vi "recombine group data.vi"(8 "error in":errorcluster, 9 "specification":T1[](array[typedef]), 10 "group in":T3, 11 "data table in":T3) -> (0 "error out":errorcluster, 2 "group out":T3, 3 "data table out":T3)   [LabVIEW 2013, in "tag bus.lvlib" / "data table.lvlib"]
doc: "Accepts a primary data table and a subgroup data table, and copies data from the group into the main table."
uses:
  data table.lvlib
  data table.ctl
  group specification.ctl
  tag/Data Type.ctl
  data polymorphs/write many/write Doubles.vi
  data polymorphs/read all/read all Doubles.vi
  data polymorphs/write many/write Singles.vi
  data polymorphs/read all/read all Singles.vi
  data polymorphs/write many/write I64s.vi
  data polymorphs/read all/read all I64s.vi
  data polymorphs/write many/write I32s.vi
  data polymorphs/read all/read all I32s.vi
  data polymorphs/write many/write I16s.vi
  data polymorphs/read all/read all I16s.vi
  data polymorphs/write many/write I8s.vi
  data polymorphs/read all/read all I8s.vi
  data polymorphs/write many/write U64s.vi
  data polymorphs/read all/read all U64s.vi
  data polymorphs/write many/write U32s.vi
  data polymorphs/read all/read all U32s.vi
  data polymorphs/write many/write U16s.vi
  data polymorphs/read all/read all U16s.vi
  data polymorphs/write many/write U8s.vi
  data polymorphs/read all/read all U8s.vi
  data polymorphs/write many/write Strings.vi
  data polymorphs/read all/read all Strings.vi
  data polymorphs/write many/write Booleans.vi
  data polymorphs/read all/read all Booleans.vi
  data polymorphs/write many/write Array of U8s.vi
  data polymorphs/read all/read all Array of U8s.vi
  data polymorphs/write many/write Array of U16s.vi
  data polymorphs/read all/read all Array of U16s.vi
  data polymorphs/write many/write Array of U32s.vi
  data polymorphs/read all/read all Array of U32s.vi
  data polymorphs/write many/write Array of U64s.vi
  data polymorphs/read all/read all Array of U64s.vi
  data polymorphs/write many/write Array of I64s.vi
  data polymorphs/read all/read all Array of I64s.vi
  data polymorphs/write many/write Array of I32s.vi
  data polymorphs/read all/read all Array of I32s.vi
  data polymorphs/write many/write Array of I16s.vi
  data polymorphs/read all/read all Array of I16s.vi
  data polymorphs/write many/write Array of I8s.vi
  data polymorphs/read all/read all Array of I8s.vi
  data polymorphs/write many/write Array of Doubles.vi
  data polymorphs/read all/read all Array of Doubles.vi
  data polymorphs/write many/write Array of Singles.vi
  data polymorphs/read all/read all Array of Singles.vi
  data polymorphs/write many/write Array of Booleans.vi
  data polymorphs/read all/read all Array of Booleans.vi
  data polymorphs/write many/write Array of Strings.vi
  data polymorphs/read all/read all Array of Strings.vi
  tag/tag descriptor.lvclass
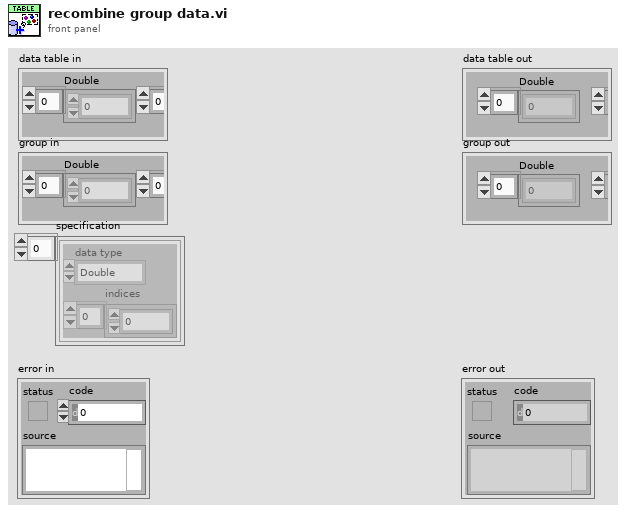
[diagram p1: front panel]
types:
  T1 = typedef "tag bus.lvlib/data table.lvlib/group specification.ctl" = cluster{"data type":T2, "indices":i32[]}
  T2 = typedef "tag bus.lvlib/tag descriptor.lvclass/Data Type.ctl" = enum16{"Double", "Single", "I64", "I32", "I16", "I8", "U64", "U32", "U16", "U8", "Boolean", "String", "Array of Double", "Array of Single", "Array of I64", "Array of I32", "Array of I16", "Array of I8", "Array of U64", "Array of U32", "Array of U16", "Array of U8", "Array of Boolean", "Array of String"}
  T3 = typedef "tag bus.lvlib/data table.lvlib/data table.ctl" = cluster{"Double":dbl[], "Single":sgl[], "I64":i64[], "I32":i32[], "I16":i16[], "I8":i8[], "U64":u64[], "U32":u32[], "U16":u16[], "U8":u8[], "Boolean":bool[], "String":string[], "Array of Double":cluster{"DBL Array":dbl[]}[], "Array of Single":cluster{"SGL Array":sgl[]}[], "Array of I64":cluster{"I64 Array":i64[]}[], "Array of I32":cluster{"I32 Array":i32[]}[], "Array of I16":cluster{"I16 Array":i16[]}[], "Array of I8":cluster{"I8 Array":i8[]}[], "Array of U64":cluster{"U64 Array":u64[]}[], "Array of U32":cluster{"U32 Array":u32[]}[], "Array of U16":cluster{"U16 Array":u16[]}[], "Array of U8":cluster{"U8 Array":u8[]}[], "Array of Boolean":cluster{"Boolean Array":bool[]}[], "Array of String":cluster{"String Array":string[]}[]}
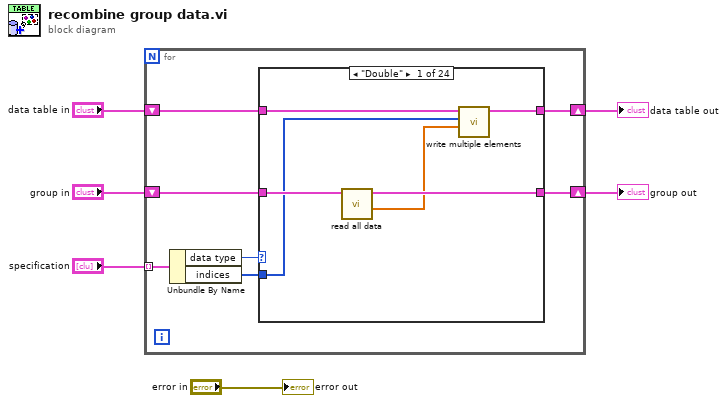
[diagram p0: block diagram]
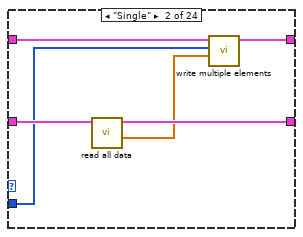
[diagram p2: hidden frame]
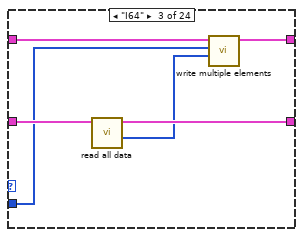
[diagram p3: hidden frame]
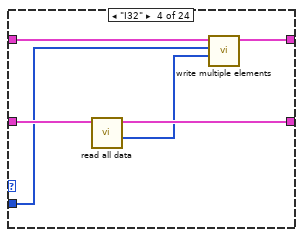
[diagram p4: hidden frame]
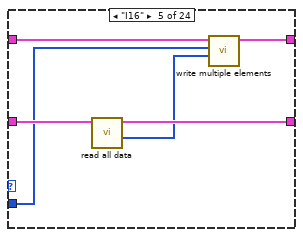
[diagram p5: hidden frame]
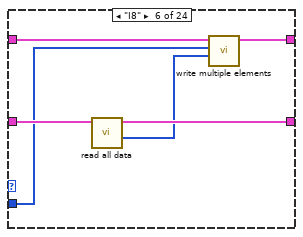
[diagram p6: hidden frame]
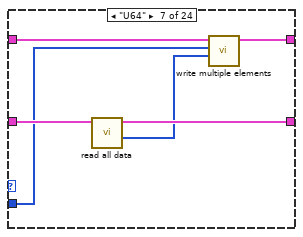
[diagram p7: hidden frame]
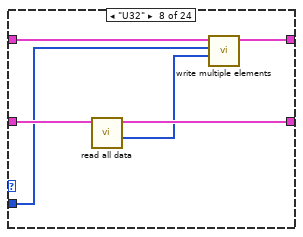
[diagram p8: hidden frame]
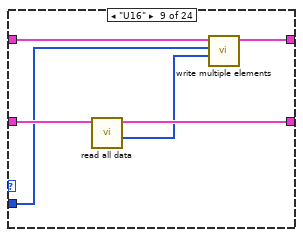
[diagram p9: hidden frame]
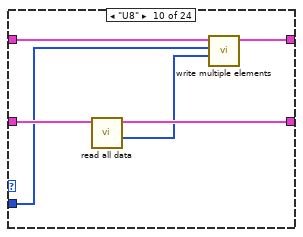
[diagram p10: hidden frame]
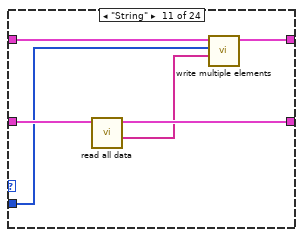
[diagram p11: hidden frame]
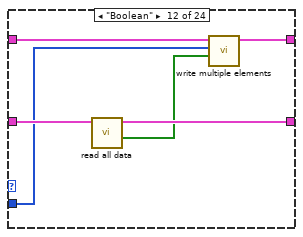
[diagram p12: hidden frame]
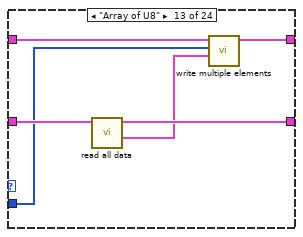
[diagram p13: hidden frame]
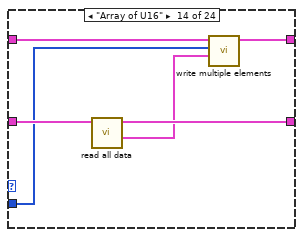
[diagram p14: hidden frame]
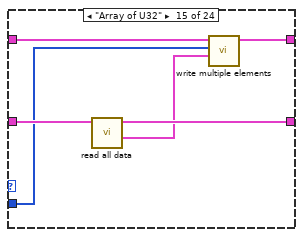
[diagram p15: hidden frame]
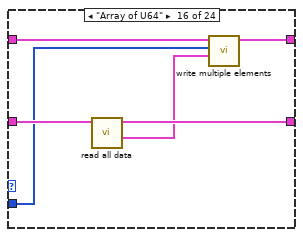
[diagram p16: hidden frame]
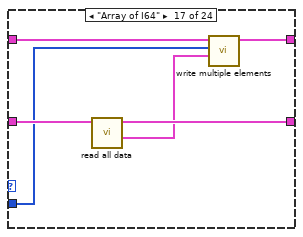
[diagram p17: hidden frame]
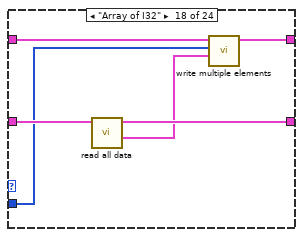
[diagram p18: hidden frame]
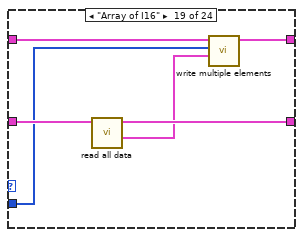
[diagram p19: hidden frame]
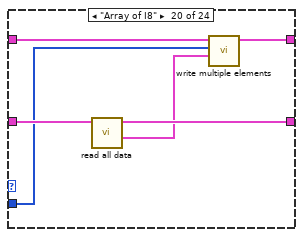
[diagram p20: hidden frame]
diagram:
  n1 = for {
    shift-right: [w9] -> w5
    shift-left: "data table in" -> [w10]
    shift-right: [w7] -> w3
    shift-left: "group in" -> [w8]
    tunnel: "specification" -> [w13] mode=indexing
    n2 = Unbundle By Name(w13) -> ("data type"=w12:T2, "indices"=w11:i32[])
    n3 = case shown="\"Double\"" w12 {
      tunnel: w11 -> [w14 w20 w26 w32 w38 w44 w50 w56 w62 w68 w74 w80 w86 w92 w98 w104 w110 w116 w122 w128 w134 w140 w146 w152]
      tunnel: w10 -> [w16 w22 w28 w34 w40 w46 w52 w58 w64 w70 w76 w82 w88 w94 w100 w106 w112 w118 w124 w130 w136 w142 w148 w154]
      tunnel: [w15 w21 w27 w33 w39 w45 w51 w57 w63 w69 w75 w81 w87 w93 w99 w105 w111 w117 w123 w129 w135 w141 w147 w153] -> w9
      tunnel: w8 -> [w19 w25 w31 w37 w43 w49 w55 w61 w67 w73 w79 w85 w91 w97 w103 w109 w115 w121 w127 w133 w139 w145 w151 w157]
      tunnel: [w18 w24 w30 w36 w42 w48 w54 w60 w66 w72 w78 w84 w90 w96 w102 w108 w114 w120 w126 w132 w138 w144 w150 w156] -> w7
      frame "Double" {
        n4 = call-poly "read all data.vi"("data table in"=w19) -> ("values"=w17:dbl[], "data table out"=w18:T3)  [unwired: 9 in]
        n5 = call-poly "write multiple elements.vi"("values"=w17, "indices"=w14, "data table in"=w16) -> ("data table out"=w15:T3)  [unwired: 8 in]
      }
      frame "Single" {
        n6 = call-poly "read all data.vi"("data table in"=w25) -> ("values"=w23:sgl[], "data table out"=w24:T3)  [unwired: 9 in]
        n7 = call-poly "write multiple elements.vi"("values"=w23, "indices"=w20, "data table in"=w22) -> ("data table out"=w21:T3)  [unwired: 8 in]
      }
      frame "I64" {
        n8 = call-poly "read all data.vi"("data table in"=w31) -> ("values"=w29:i64[], "data table out"=w30:T3)  [unwired: 9 in]
        n9 = call-poly "write multiple elements.vi"("values"=w29, "indices"=w26, "data table in"=w28) -> ("data table out"=w27:T3)  [unwired: 8 in]
      }
      frame "I32" {
        n10 = call-poly "read all data.vi"("data table in"=w37) -> ("values"=w35:i32[], "data table out"=w36:T3)  [unwired: 9 in]
        n11 = call-poly "write multiple elements.vi"("values"=w35, "indices"=w32, "data table in"=w34) -> ("data table out"=w33:T3)  [unwired: 8 in]
      }
      frame "I16" {
        n12 = call-poly "read all data.vi"("data table in"=w43) -> ("values"=w41:i16[], "data table out"=w42:T3)  [unwired: 9 in]
        n13 = call-poly "write multiple elements.vi"("values"=w41, "indices"=w38, "data table in"=w40) -> ("data table out"=w39:T3)  [unwired: 8 in]
      }
      frame "I8" {
        n14 = call-poly "read all data.vi"("data table in"=w49) -> ("values"=w47:i8[], "data table out"=w48:T3)  [unwired: 9 in]
        n15 = call-poly "write multiple elements.vi"("values"=w47, "indices"=w44, "data table in"=w46) -> ("data table out"=w45:T3)  [unwired: 8 in]
      }
      frame "U64" {
        n16 = call-poly "read all data.vi"("data table in"=w55) -> ("values"=w53:u64[], "data table out"=w54:T3)  [unwired: 9 in]
        n17 = call-poly "write multiple elements.vi"("values"=w53, "indices"=w50, "data table in"=w52) -> ("data table out"=w51:T3)  [unwired: 8 in]
      }
      frame "U32" {
        n18 = call-poly "read all data.vi"("data table in"=w61) -> ("values"=w59:u32[], "data table out"=w60:T3)  [unwired: 9 in]
        n19 = call-poly "write multiple elements.vi"("values"=w59, "indices"=w56, "data table in"=w58) -> ("data table out"=w57:T3)  [unwired: 8 in]
      }
      frame "U16" {
        n20 = call-poly "read all data.vi"("data table in"=w67) -> ("values"=w65:u16[], "data table out"=w66:T3)  [unwired: 9 in]
        n21 = call-poly "write multiple elements.vi"("values"=w65, "indices"=w62, "data table in"=w64) -> ("data table out"=w63:T3)  [unwired: 8 in]
      }
      frame "U8" {
        n22 = call-poly "read all data.vi"("data table in"=w73) -> ("values"=w71:u8[], "data table out"=w72:T3)  [unwired: 9 in]
        n23 = call-poly "write multiple elements.vi"("values"=w71, "indices"=w68, "data table in"=w70) -> ("data table out"=w69:T3)  [unwired: 8 in]
      }
      frame "String" {
        n24 = call-poly "read all data.vi"("data table in"=w79) -> ("values"=w77:string[], "data table out"=w78:T3)  [unwired: 9 in]
        n25 = call-poly "write multiple elements.vi"("values"=w77, "indices"=w74, "data table in"=w76) -> ("data table out"=w75:T3)  [unwired: 8 in]
      }
      frame "Boolean" {
        n26 = call-poly "read all data.vi"("data table in"=w85) -> ("values"=w83:bool[], "data table out"=w84:T3)  [unwired: 9 in]
        n27 = call-poly "write multiple elements.vi"("values"=w83, "indices"=w80, "data table in"=w82) -> ("data table out"=w81:T3)  [unwired: 8 in]
      }
      frame "Array of U8" {
        n28 = call-poly "read all data.vi"("data table in"=w91) -> ("values"=w89:cluster{"U8 Array":u8[]}[], "data table out"=w90:T3)  [unwired: 9 in]
        n29 = call-poly "write multiple elements.vi"("values"=w89, "indices"=w86, "data table in"=w88) -> ("data table out"=w87:T3)  [unwired: 8 in]
      }
      frame "Array of U16" {
        n30 = call-poly "read all data.vi"("data table in"=w97) -> ("values"=w95:cluster{"Array":u16[]}[], "data table out"=w96:T3)  [unwired: 9 in]
        n31 = call-poly "write multiple elements.vi"("values"=w95, "indices"=w92, "data table in"=w94) -> ("data table out"=w93:T3)  [unwired: 8 in]
      }
      frame "Array of U32" {
        n32 = call-poly "read all data.vi"("data table in"=w103) -> ("values"=w101:cluster{"Array":u32[]}[], "data table out"=w102:T3)  [unwired: 9 in]
        n33 = call-poly "write multiple elements.vi"("values"=w101, "indices"=w98, "data table in"=w100) -> ("data table out"=w99:T3)  [unwired: 8 in]
      }
      frame "Array of U64" {
        n34 = call-poly "read all data.vi"("data table in"=w109) -> ("values"=w107:cluster{"Array":u64[]}[], "data table out"=w108:T3)  [unwired: 9 in]
        n35 = call-poly "write multiple elements.vi"("values"=w107, "indices"=w104, "data table in"=w106) -> ("data table out"=w105:T3)  [unwired: 8 in]
      }
      frame "Array of I64" {
        n36 = call-poly "read all data.vi"("data table in"=w115) -> ("values"=w113:cluster{"Array":i64[]}[], "data table out"=w114:T3)  [unwired: 9 in]
        n37 = call-poly "write multiple elements.vi"("values"=w113, "indices"=w110, "data table in"=w112) -> ("data table out"=w111:T3)  [unwired: 8 in]
      }
      frame "Array of I32" {
        n38 = call-poly "read all data.vi"("data table in"=w121) -> ("values"=w119:cluster{"Array":i32[]}[], "data table out"=w120:T3)  [unwired: 9 in]
        n39 = call-poly "write multiple elements.vi"("values"=w119, "indices"=w116, "data table in"=w118) -> ("data table out"=w117:T3)  [unwired: 8 in]
      }
      frame "Array of I16" {
        n40 = call-poly "read all data.vi"("data table in"=w127) -> ("values"=w125:cluster{"Array":i16[]}[], "data table out"=w126:T3)  [unwired: 9 in]
        n41 = call-poly "write multiple elements.vi"("values"=w125, "indices"=w122, "data table in"=w124) -> ("data table out"=w123:T3)  [unwired: 8 in]
      }
      frame "Array of I8" {
        n42 = call-poly "read all data.vi"("data table in"=w133) -> ("values"=w131:cluster{"Array":i8[]}[], "data table out"=w132:T3)  [unwired: 9 in]
        n43 = call-poly "write multiple elements.vi"("values"=w131, "indices"=w128, "data table in"=w130) -> ("data table out"=w129:T3)  [unwired: 8 in]
      }
      frame "Array of Double" {
        n44 = call-poly "read all data.vi"("data table in"=w139) -> ("values"=w137:cluster{"Array":dbl[]}[], "data table out"=w138:T3)  [unwired: 9 in]
        n45 = call-poly "write multiple elements.vi"("values"=w137, "indices"=w134, "data table in"=w136) -> ("data table out"=w135:T3)  [unwired: 8 in]
      }
      frame "Array of Single" {
        n46 = call-poly "read all data.vi"("data table in"=w145) -> ("values"=w143:cluster{"Array":sgl[]}[], "data table out"=w144:T3)  [unwired: 9 in]
        n47 = call-poly "write multiple elements.vi"("values"=w143, "indices"=w140, "data table in"=w142) -> ("data table out"=w141:T3)  [unwired: 8 in]
      }
      frame "Array of Boolean" {
        n48 = call-poly "read all data.vi"("data table in"=w151) -> ("values"=w149:cluster{"Array":bool[]}[], "data table out"=w150:T3)  [unwired: 9 in]
        n49 = call-poly "write multiple elements.vi"("values"=w149, "indices"=w146, "data table in"=w148) -> ("data table out"=w147:T3)  [unwired: 8 in]
      }
      frame "Array of String" {
        n50 = call-poly "read all data.vi"("data table in"=w157) -> ("values"=w155:cluster{"Array":string[]}[], "data table out"=w156:T3)  [unwired: 9 in]
        n51 = call-poly "write multiple elements.vi"("values"=w155, "indices"=w152, "data table in"=w154) -> ("data table out"=w153:T3)  [unwired: 8 in]
      }
    }
  }
  "data table out" <- w5
  "group out" <- w3
  "error out" <- "error in"
